vi "getRunId.vi"(8 "error in (no error)":errorcluster, 11 "HWController in":refnum<class "HWController.lvclass">) -> (0 "error out":errorcluster, 2 "Numeric":i32, 3 "HWController out":refnum<class "HWController.lvclass">)   [LabVIEW 2009, in "Hardware.lvlib" / "HWControllers.lvlib" / "HWController.lvclass"]
uses:
  HWController.lvclass
  HWController.lvclass/HWController.ctl
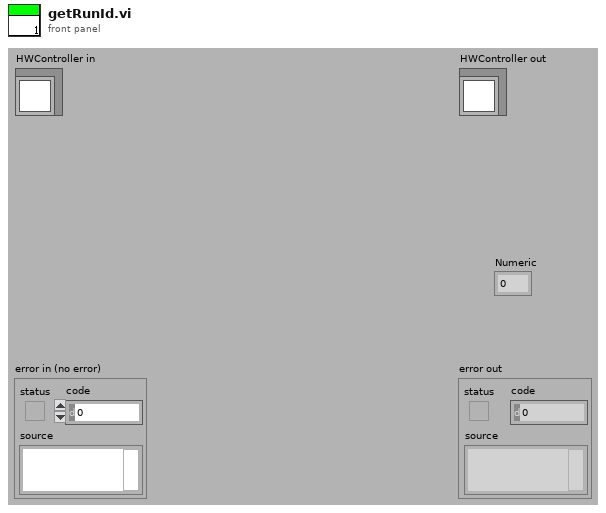
[diagram p1: front panel]
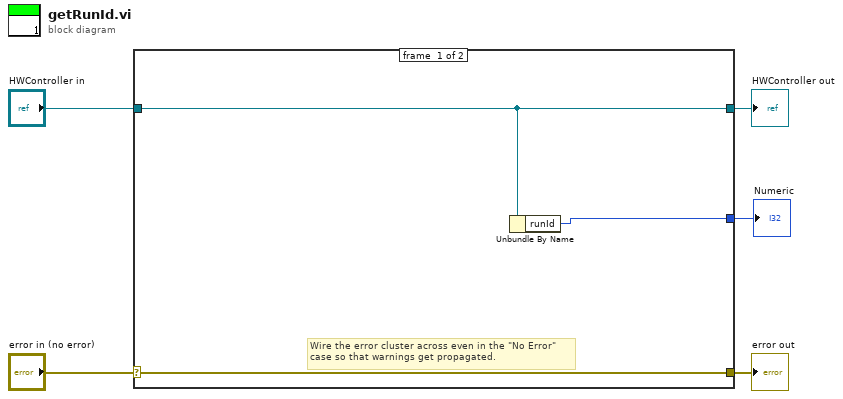
[diagram p0: block diagram]
diagram:
  n1 = case shown="No Error" "error in (no error)" {
    selector: "error in (no error)" -> [w8 w10]
    tunnel: [w8 w10] -> w4
    tunnel: [w7 w9] -> w2
    tunnel: "HWController in" -> [w7 w9]
    tunnel: [w6 _] -> w1
    frame #0 {
      # "Wire the error cluster across even in the \"No Error\"\ncase so that warnings get propagated."
      n2 = Unbundle By Name(w7) -> ("runId"=w6:i32)
    }
    frame #1 {
    }
  }
  "error out" <- w4
  "HWController out" <- w2
  "Numeric" <- w1
